vi "h5_write_xywav.vi"(7 "dataset name":string, 8 "error in":errorcluster, 10 "xywave":T1={"attributes"=variant, "Z"={"data"=[], "units"="au"}, "X"={"start"=0.0, "delta"=1.0, "units"="index", "dim"="x"}, "Y"={"start"=0.0, "delta"=1.0, "units"="index", "dim"="y"}}, 11 "h5 ref in":T2 format="%.0x") -> (0 "error out":errorcluster, 2 "dup xywave":T1={"attributes"=variant, "Z"={"data"=[], "units"="au"}, "X"={"start"=0.0, "delta"=1.0, "units"="index", "dim"="x"}, "Y"={"start"=0.0, "delta"=1.0, "units"="index", "dim"="y"}}, 3 "dup h5 ref":T2 format="%.0x")   [LabVIEW 2015]
uses:
  <vilib>/addons/h5labview2/base/hid_t.ctl
  xwave/xywav.ctl
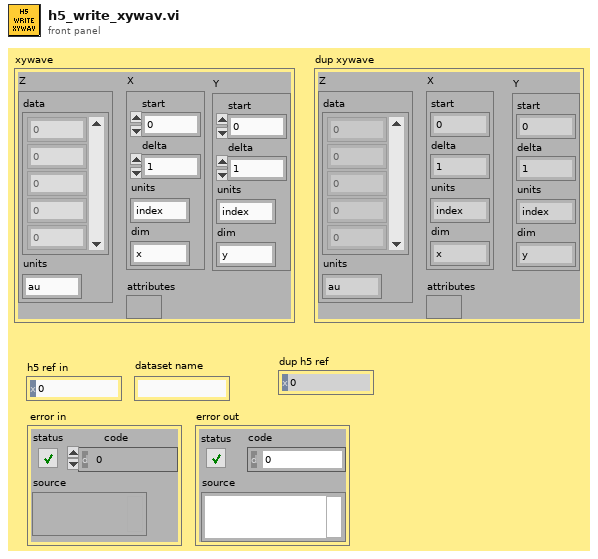
[diagram p1: front panel]
types:
  T1 = typedef "xywav.ctl" = cluster{"attributes":variant, "Z":cluster{"data":dbl[][], "units":string}, "X":cluster{"start":dbl, "delta":dbl, "units":string, "dim":string}, "Y":cluster{"start":dbl, "delta":dbl, "units":string, "dim":string}}
  T2 = typedef "hid_t.ctl" = i32
  T3 = cluster{"x0":dbl, "dx":dbl, "y0":dbl, "dy":dbl, "x units":string, "y units":string}
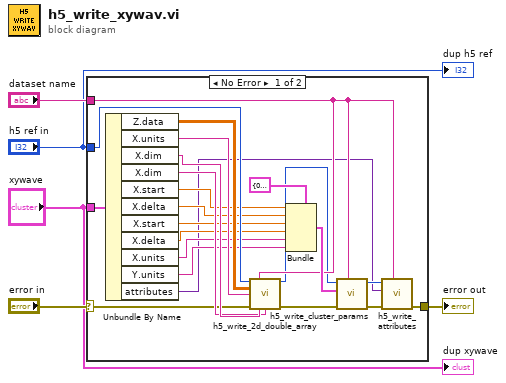
[diagram p0: block diagram]
diagram:
  n1 = case shown="No Error" "error in" {
    selector: "error in" -> [w16 w28]
    tunnel: [w22 w28] -> w5
    tunnel: "h5 ref in" -> [w17 _]
    tunnel: "xywave" -> [w27 _]
    tunnel: "dataset name" -> [w18 _]
    frame No Error {
      n2 = Unbundle By Name(w27) -> ("Z.data"=w15:dbl[][], "X.units"=w21:string, "X.dim"=w20:string, "X.dim"=w19:string, "X.start"=w14:dbl, "X.delta"=w13:dbl, "X.start"=w12:dbl, "X.delta"=w11:dbl, "X.units"=w10:string, "Y.units"=w9:string, "attributes"=w6:variant)
      n3 = call "h5_write_2d_double_array.vi"("h5 dir ref"=w17, "dataset name"=w18, "array"=w15, "units (au)"=w21, "error in (no error)"=w16, "dim1 (index)"=w20, "dim2 (index)"=w19) -> ("h5 obj ref"=w7:i32, "error out"=w8:errorcluster)  [unwired: 7 in]
      n4 = Bundle(cluster=T3 {"x0"=0.0, "dx"=0.0, "y0"=0.0, "dy"=0.0, "x units"="", "y units"=""} ("xwave"), "x0"=w14, "dx"=w13, "y0"=w12, "dy"=w11, "x units"=w10, "y units"=w9) -> (w25:T3)
      n5 = call "h5_write_cluster_params.vi"("object name"=w18, "error in (no error)"=w8, "cluster"=w25, "h5 obj ref"=w7) -> ("error out"=w24:errorcluster, "h5 obj ref"=w23:T2)  [unwired: 6 in]
      n6 = call "h5_write_attributes.vi"("object name"=w18, "error in"=w24, "attributes"=w6, "h5 ref"=w23) -> ("error out"=w22:errorcluster)  [unwired: 6 in, 1 out]
    }
    frame Error {
    }
  }
  "error out" <- w5
  "dup h5 ref" <- "h5 ref in"
  "dup xywave" <- "xywave"
